vi "Revision Query.vi"(8 "error in (no error)":errorcluster, 11 "VISA resource name":refnum<visa-resource-name>) -> (0 "error out":errorcluster, 1 "Instrument Firmware Revision":string, 2 "Instrument Driver Revision":string, 3 "VISA resource name out":refnum<visa-resource-name>)   [LabVIEW 2020, in "Agilent 34405.lvlib"]
doc: "Queries the current instrument firmware revision and instrument driver revision.\n\nRefer to the Readme file for detailed driver information including modification history."
uses:
  <instrlib>/Agilent 34405/Agilent 34405.lvlib
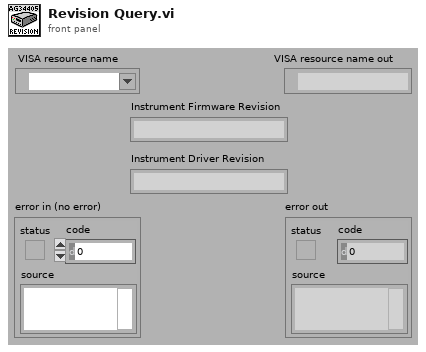
[diagram p1: front panel]
types:
  T1 = enum32{"invalid app kind", "Development System", "Run Time System", "Student Edition", "Embedded LabVIEW", "Evaluation", "Custom"}
  T2 = cluster{"Major":u16, "Minor":u16, "Fix":u16, "Build":u16}
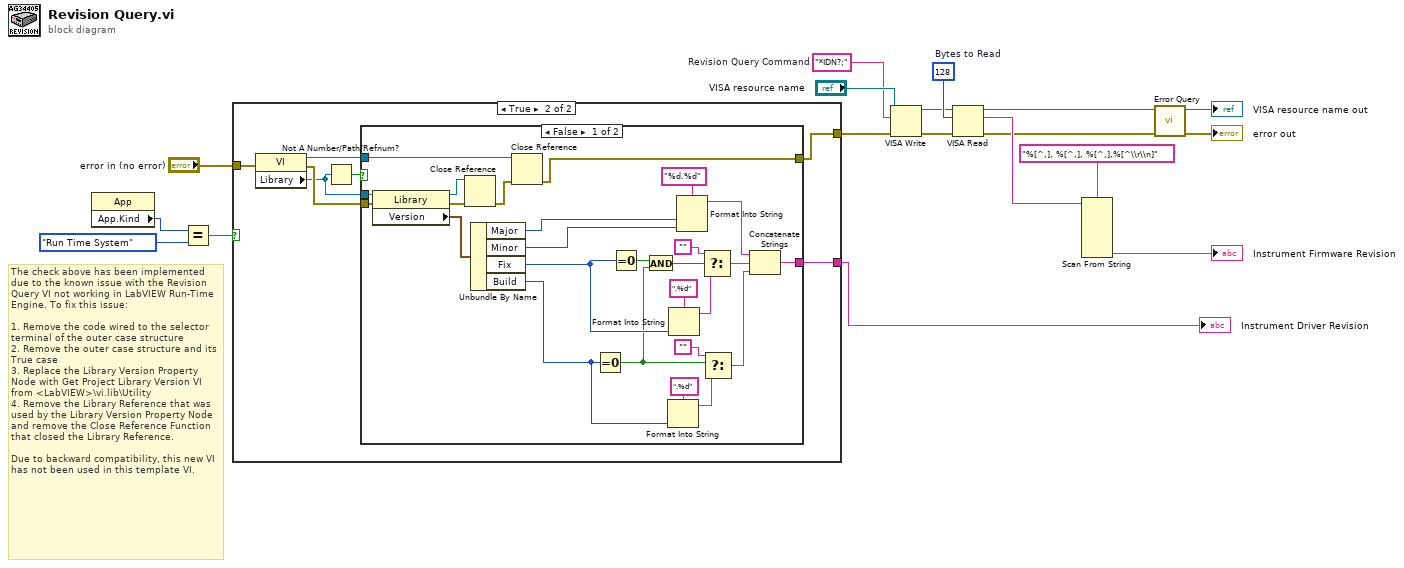
[diagram p0: block diagram]
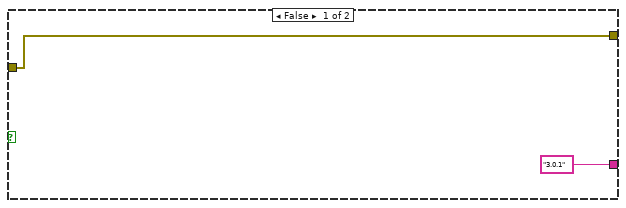
[diagram p2: hidden frame]
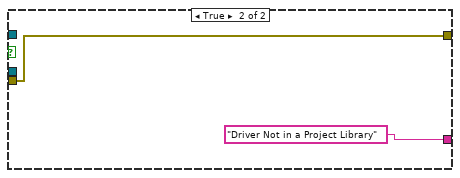
[diagram p3: hidden frame]
diagram:
  w13 = "*IDN?;"  # Revision Query Command
  w16 = u32 128  # Bytes to Read
  # "The check above has been implemented due to the known issue with the Revision Query VI not working in LabVIEW Run-Time Engine. To fix this issue:\n\n1. Remove the code wired to the selector terminal of the outer case structure\n2. Remove the outer case structure and its True case\n3. Replace the Library Version Property Node with Get Project Library Version VI from <LabVIEW>\\vi.lib\\Utility\n4. Remove the Library Reference that was used by the Library Version Property Node and remove the Close Reference Function that closed the Library Reference.\n\nDue to backward compatibility, this new VI has not been used in this template VI."
  n1 = property on="Property Node" class="App"() -> ("App.Kind"=w3:T1)  [unwired: 2 in, 2 out]
  n2 = Equal?(x=w3, y=T1."Run Time System" ("Application:Kind")) -> (x = y?=w1:bool)
  n3 = case shown="True" w1 {
    tunnel: ["3.0.1" w23] -> w6
    tunnel: "error in (no error)" -> [w20 w22]
    tunnel: [w20 w21] -> w4
    frame False {
    }
    frame True {
      n4 = property on="Property Node" class="VI"(error in=w22) -> (reference out=w27:refnum<vi>, error out=w26:errorcluster, "Library"=w25:refnum<vi>)  [unwired: 1 in]
      n5 = Not A Number/Path/Refnum?(number/path/refnum=w25) -> (NaN/Path/Refnum?=w24:bool)
      n6 = case shown="False" w24 {
        tunnel: w27 -> [w50 _]
        tunnel: w26 -> [w37 w55]
        tunnel: [w32 w55] -> w21
        tunnel: [w31 "Driver Not in a Project Library"] -> w23
        tunnel: w25 -> [w30 _]
        frame False {
          n7 = property on="Property Node" class="Library"(reference=w30, error in=w37) -> (reference out=w52:refnum<vi>, error out=w53:errorcluster, "Version"=w49:T2)
          n8 = Close Reference(reference=w52, error in (no error)=w53) -> (error out=w51:errorcluster)
          n9 = Unbundle By Name(w49) -> ("Major"=w40:u16, "Minor"=w39:u16, "Fix"=w36:u16, "Build"=w38:u16)
          n10 = Close Reference(reference=w50, error in (no error)=w51) -> (error out=w32:errorcluster)
          n11 = Equal To 0?(x=w38) -> (x = 0?=w34:bool)
          n12 = Equal To 0?(x=w36) -> (x = 0?=w35:bool)
          n13 = And(x=w35, y=w34) -> (x .and. y?=w33:bool)
          n14 = Format Into String(format string=".%d", w38) -> (resulting string=w43:string)  [unwired: 2 in, 1 out]
          n15 = Format Into String(format string=".%d", w36) -> (resulting string=w47:string)  [unwired: 2 in, 1 out]
          n16 = Format Into String(format string="%d.%d", w40, w39) -> (resulting string=w45:string)  [unwired: 2 in, 1 out]
          n17 = Select(t="" ("Empty String Constant"), s=w33, f=w47) -> (s? t:f=w44:string)
          n18 = Select(t="" ("Empty String Constant"), s=w34, f=w43) -> (s? t:f=w41:string)
          n19 = Concatenate Strings(w45, w44, w41) -> (w31:string)
        }
        frame True {
        }
      }
    }
  }
  "Instrument Driver Revision" <- w6
  n20 = VISA Write(VISA resource name="VISA resource name", write buffer=w13, error in (no error)=w4) -> (VISA resource name out=w15:refnum<visa-resource-name>, error out=w14:errorcluster)  [unwired: 1 out]
  n21 = VISA Read(VISA resource name=w15, byte count=w16, error in (no error)=w14) -> (VISA resource name out=w9:refnum<visa-resource-name>, read buffer=w12:string, error out=w10:errorcluster)  [unwired: 1 out]
  n22 = Scan From String(format string="%[^,], %[^,], %[^,],%[^\\r\\n]", input string=w12) -> (output 4=→"Instrument Firmware Revision":string)  [unwired: 2 in, 10 out]
  n23 = call <instrlib>:"Error Query.vi"("error in (no error)"=w10, "VISA resource name"=w9) -> ("error out"=→"error out":errorcluster, "VISA resource name out"=→"VISA resource name out":refnum<visa-resource-name>)  [unwired: 8 out]
